vi "Create Plugin Template.vi"(0 "Project Path":path=path "D:/Reference Architecture/Test.lvproj", 5 "Description":string, 11 "error in (no error)":errorcluster) -> (15 "error out":errorcluster)   [LabVIEW 2021, in "Migrator.lvlib"]
uses:
  Migrator.lvlib
  Measurement Plugin Generator/_Editor/MeasurementService Editor.lvlib
  Migrator Reusables/Migrator Reusables.lvlib
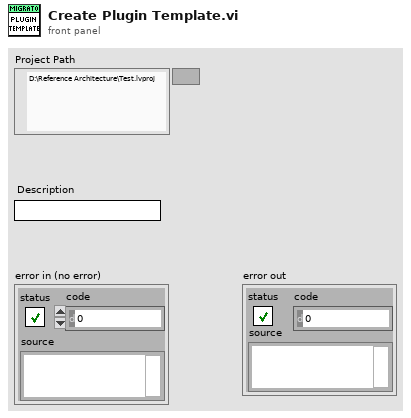
[diagram p1: front panel]
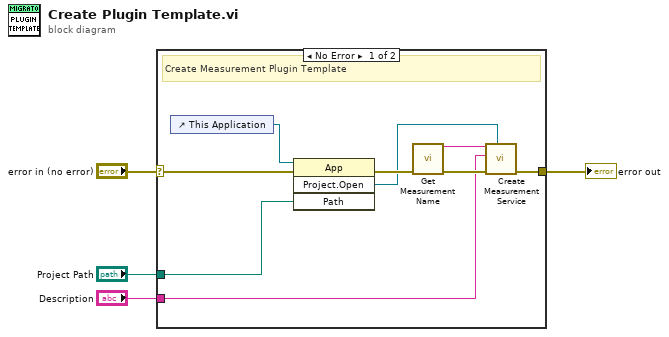
[diagram p0: block diagram]
diagram:
  n1 = case shown="No Error" "error in (no error)" {
    selector: "error in (no error)" -> [w8 w14]
    tunnel: "Project Path" -> [w7 _]
    tunnel: [w10 w14] -> w2
    tunnel: "Description" -> [w11 _]
    frame No Error {
      # "Create Measurement Plugin Template"
      n2 = control-ref of="This Application"() -> (w9:refnum<vi>)
      n3 = invoke class="App" method="Project.Open"(reference=w9, error in=w8, "Path"=w7) -> (error out=w6:errorcluster, "Project:Open"=w5:refnum<vi>)  [unwired: 1 in, 2 out]
      n4 = call "Get Measurement Name.vi"("error in (no error)"=w6) -> ("Name Out"=w12:string, "error out"=w13:errorcluster)  [unwired: 13 in]
      n5 = call "Create Measurement Service.vi"("project ref"=w5, "error in (no error)"=w13, "measurement plug-in description"=w11, "measurement plug-in name"=w12) -> ("error out"=w10:errorcluster)  [unwired: 7 in]
    }
    frame Error {
    }
  }
  "error out" <- w2
